vi "CheckMultiLine.vi"(11 "Code":string) -> (3 "MultiLine?":bool)   [LabVIEW 2020]
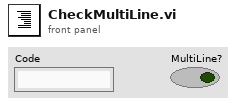
[diagram p1: front panel]
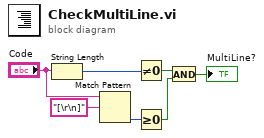
[diagram p0: block diagram]
diagram:
  n1 = String Length(string="Code") -> (length=w1:i32)
  n2 = Match Pattern(string="Code", regular expression="[\r\n]") -> (offset past match=w4:i32)  [unwired: 1 in, 3 out]
  n3 = Not Equal To 0?(x=w1) -> (x != 0?=w5:bool)
  n4 = Greater Or Equal To 0?(x=w4) -> (x >= 0?=w6:bool)
  n5 = And(x=w5, y=w6) -> (x .and. y?=→"MultiLine?":bool)
